vi "Psychrmoetric Chart by DP.vi"() -> (0 "Psych Chart by DP":dbl[][](array[numeric]))   [LabVIEW 2020]
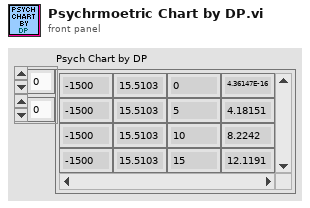
[diagram p1: front panel]
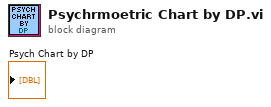
[diagram p0: block diagram]
diagram:
